vi "PR Tags.vi"(11 "PR Module Configs":T1[](array[typedef]) {"Settings"."PID 2 Parameters"."output range"."output low" format="%.2f"; "Settings"."PID 2 Parameters"."output range"."output high" min=0.0 max=100.0 format="%.2f"; "Settings"."PID 2 Parameters"."PID gains"."derivative time (Td, min)" format="%.3f"; "Settings"."PID 2 Parameters"."PID gains"."integral time (Ti, min)" format="%.3f"; "Settings"."PID 2 Parameters"."PID gains"."proportional gain (Kc)" format="%.3f"}) -> (1 "PID 2 Out Tag 2":string, 2 "All  Numeric Tags 6":string[](array[string]), 3 "All Boolean Tags 6":string[](array[string]), 4 "PR Module Tags Array":T6[](array[typedef]), 5 "4-20mA Module Tag Names":T6)   [LabVIEW 2018]
uses:
  Pressure Regulator Control Module/Pressure Regulator/Controls/4-20mA Module Tag Names Cluster.ctl
  Pressure Regulator Control Module/Pressure Regulator/Controls/4-20mA Module Config Cluster.ctl
  <vilib>/Utility/miscctls.llb/LVPoint32TypeDef.ctl
  Pressure Regulator Control Module/Pressure Regulator/Controls/4-20mA Module Settings Cluster.ctl
  Pressure Transmitter/Pressure Transmitter Device Settings.ctl
  Pressure Reg Module/Pressure Regulator Device Settings.ctl
  Pressure Regulator Control Module/Pressure Regulator/4-20mA Module.lvlib
  Pressure Transmitter/Pressure Transmitter Library.lvlib
  Pressure Reg Module/Pressure Regulator Library.lvlib
panel:
  # "Instrument Settings"
  # "Instrument Settings"
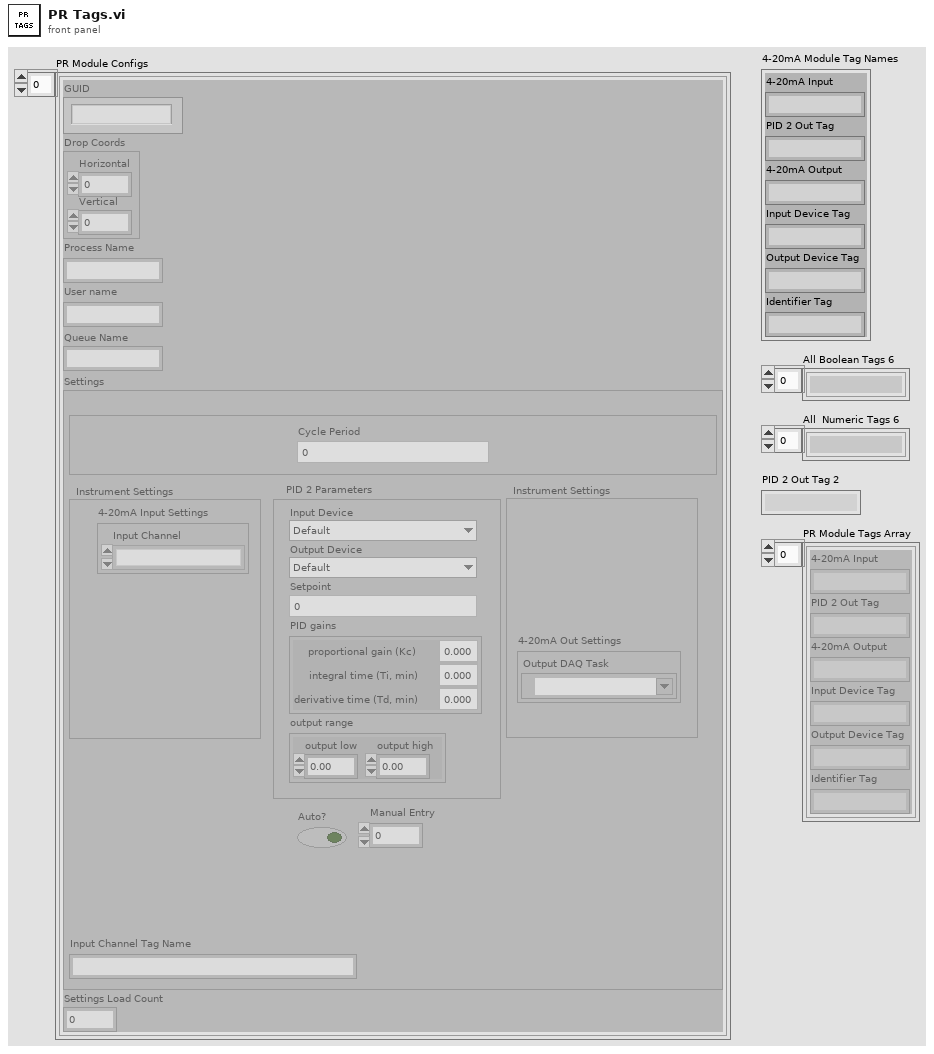
[diagram p1: front panel]
types:
  T1 = typedef "4-20mA Module.lvlib/4-20mA Module Config Cluster.ctl" = cluster{"GUID":string, "Drop Coords":T2, "Process Name":string, "User name":string, "Queue Name":string, "Settings":T3, "Settings Load Count":i32}
  T2 = typedef "LVPoint32TypeDef.ctl" = cluster{"Horizontal":i32, "Vertical":i32}
  T3 = typedef "4-20mA Module.lvlib/4-20mA Module Settings Cluster.ctl" = cluster{"Cycle Period":dbl, "PID 2 Parameters":cluster{"Input Device":enum16{"Default", "4-20mA"}, "Output Device":enum16{"Default", "Equilibar Pressure Reg", "Flow Regulator"}, "Setpoint":dbl, "PID gains":cluster{"proportional gain (Kc)":dbl, "integral time (Ti, min)":dbl, "derivative time (Td, min)":dbl}, "output range":cluster{"output low":dbl, "output high":dbl}}, "Manual Entry":dbl, "Auto?":bool, "4-20mA Input Settings":T4, "4-20mA Out Settings":T5, "Input Channel Tag Name ":string}
  T4 = typedef "Pressure Transmitter Library.lvlib/Pressure Transmitter Device Settings.ctl" = cluster{"Input Channel ":u16}
  T5 = typedef "Pressure Regulator Library.lvlib/Pressure Regulator Device Settings.ctl" = cluster{"Output DAQ Task":refnum<k21>}
  T6 = typedef "4-20mA Module.lvlib/4-20mA Module Tag Names Cluster.ctl" = cluster{"4-20mA Input":string, "PID 2 Out Tag":string, "4-20mA Output":string, "Input Device Tag":string, "Output Device Tag":string, "Identifier Tag":string}
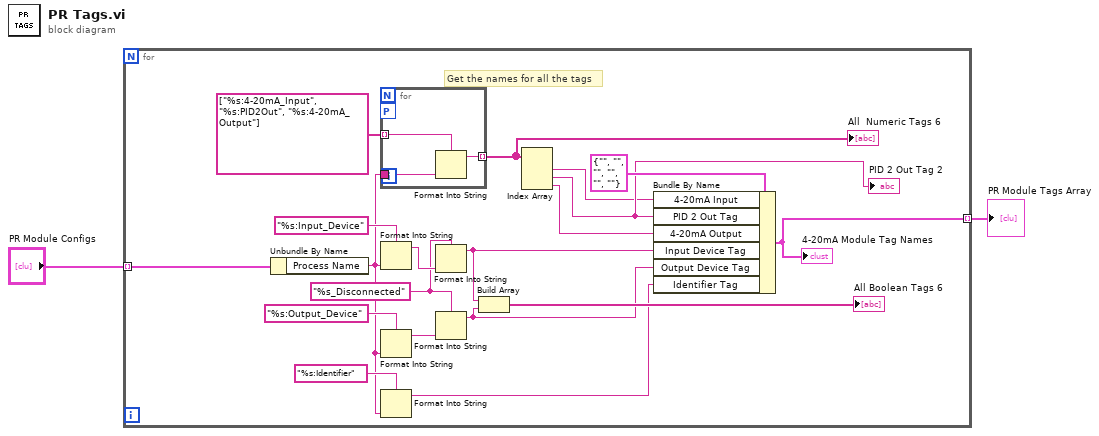
[diagram p0: block diagram]
diagram:
  n1 = for {
    tunnel: "PR Module Configs" -> [w7] mode=indexing
    tunnel: [w6] -> w2 mode=indexing
    w8 = "%s_Disconnected"
    # "Get the names for all the tags"
    n2 = Unbundle By Name(w7) -> ("Process Name"=w4:string)
    n3 = for {
      tunnel: string[] ["%s:4-20mA_Input", "%s:PID2Out", "%s:4-20mA_Output"] -> [w24] mode=indexing
      tunnel: w4 -> [w23]
      tunnel: [w22] -> w12 mode=indexing
      workers-P: _ -> [_]
      n4 = Format Into String(format string=w24, w23) -> (resulting string=w22:string)  [unwired: 2 in, 1 out]
    }
    "All  Numeric Tags 6" <- w12
    n5 = Format Into String(format string="%s:Input_Device", w4) -> (resulting string=w20:string)  [unwired: 2 in, 1 out]
    n6 = Format Into String(format string="%s:Output_Device", w4) -> (resulting string=w19:string)  [unwired: 2 in, 1 out]
    n7 = Format Into String(format string="%s:Identifier", w4) -> (resulting string=w3:string)  [unwired: 2 in, 1 out]
    n8 = Format Into String(format string=w8, w20) -> (resulting string=w14:string)  [unwired: 2 in, 1 out]
    n9 = Format Into String(format string=w8, w19) -> (resulting string=w13:string)  [unwired: 2 in, 1 out]
    n10 = Build Array(w14, w13) -> (→"All Boolean Tags 6":string[])
    n11 = Index Array(array=w12) -> (element #1=w10:string, element #2=w11:string, element #3=w9:string)  [unwired: 3 in]
    "PID 2 Out Tag 2" <- w11
    n12 = Bundle By Name(cluster=T6 {"4-20mA Input"="", "PID 2 Out Tag"="", "4-20mA Output"="", "Input Device Tag"="", "Output Device Tag"="", "Identifier Tag"=""} ("Feed Module Tag Names"), "4-20mA Input"=w10, "PID 2 Out Tag"=w11, "4-20mA Output"=w9, "Input Device Tag"=w14, "Output Device Tag"=w13, "Identifier Tag"=w3) -> (w6:T6)
    "4-20mA Module Tag Names" <- w6
  }
  "PR Module Tags Array" <- w2
